vi "ScaleGenCtrl.vi"(6 "Scale Dir":T1=enum."Full scale -> Model scale", 8 "Scale factor":dbl, 11 "Gen Control (In)":T2) -> (3 "Gen Control (Out)":T2)   [LabVIEW 2018]
uses:
  Clusters/GenCtrl.ctl
  Clusters/GenMode.ctl
  Clusters/ScalingEnum.ctl
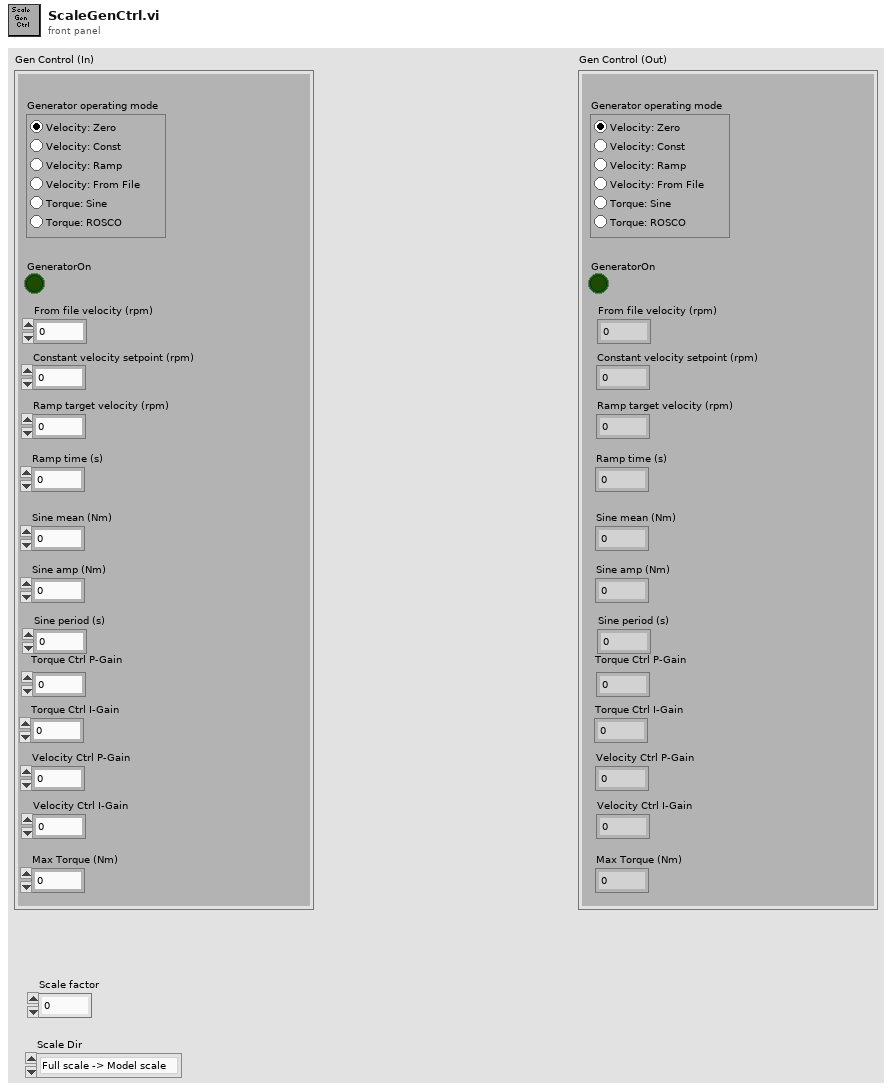
[diagram p1: front panel]
types:
  T1 = typedef "ScalingEnum.ctl" = enum16{"Model scale -> Full scale", "Full scale -> Model scale"}
  T2 = typedef "GenCtrl.ctl" = cluster{"Constant velocity setpoint (rpm)":dbl, "Ramp target velocity (rpm)":dbl, "Ramp time (s)":dbl, "Sine mean (Nm)":dbl, "Sine amp (Nm)":dbl, "Sine period (s)":dbl, "Torque Ctrl I-Gain":dbl, "Velocity Ctrl P-Gain":dbl, "Velocity Ctrl I-Gain":dbl, "Max Torque (Nm)":dbl, "GeneratorOn":bool, "Torque Ctrl P-Gain":dbl, "From file velocity (rpm)":dbl, "Generator operating mode":T3}
  T3 = typedef "GenMode.ctl" = enum32{"Velocity: Zero", "Velocity: Const.", "Velocity: Ramp", "Velocity: From File", "Torque: Sine", "Torque: ROSCO"}
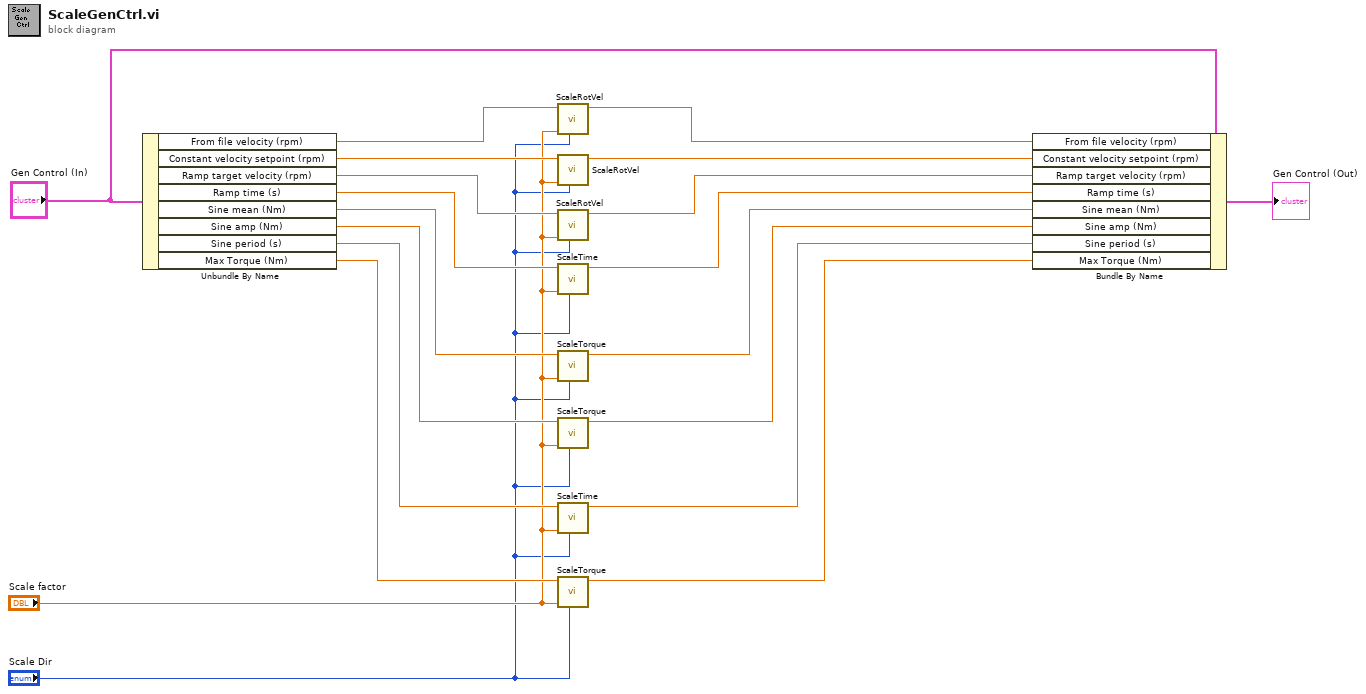
[diagram p0: block diagram]
diagram:
  n1 = Unbundle By Name("Gen Control (In)") -> ("From file velocity (rpm)"=w4:dbl, "Constant velocity setpoint (rpm)"=w18:dbl, "Ramp target velocity (rpm)"=w17:dbl, "Ramp time (s)"=w16:dbl, "Sine mean (Nm)"=w12:dbl, "Sine amp (Nm)"=w10:dbl, "Sine period (s)"=w8:dbl, "Max Torque (Nm)"=w6:dbl)
  n2 = call "ScaleRotVel.vi"("Scale Dir"="Scale Dir", "Scale factor"="Scale factor", "Rotational Velocity (In)"=w4) -> ("Rotational Velocity (Out)"=w3:dbl)  [unwired: 8 in]
  n3 = call "ScaleRotVel.vi"("Scale Dir"="Scale Dir", "Scale factor"="Scale factor", "Rotational Velocity (In)"=w18) -> ("Rotational Velocity (Out)"=w15:dbl)  [unwired: 8 in]
  n4 = call "ScaleRotVel.vi"("Scale Dir"="Scale Dir", "Scale factor"="Scale factor", "Rotational Velocity (In)"=w17) -> ("Rotational Velocity (Out)"=w14:dbl)  [unwired: 8 in]
  n5 = call "ScaleTime.vi"("Scale Dir"="Scale Dir", "Scale factor"="Scale factor", "Time (In)"=w16) -> ("Time OUT (Out)"=w13:dbl)  [unwired: 8 in]
  n6 = call "ScaleTorque.vi"("Scale Dir"="Scale Dir", "Scale factor"="Scale factor", "Torque (In)"=w12) -> ("Torque (Out)"=w11:dbl)  [unwired: 8 in]
  n7 = call "ScaleTorque.vi"("Scale Dir"="Scale Dir", "Scale factor"="Scale factor", "Torque (In)"=w10) -> ("Torque (Out)"=w9:dbl)  [unwired: 8 in]
  n8 = call "ScaleTime.vi"("Scale Dir"="Scale Dir", "Scale factor"="Scale factor", "Time (In)"=w8) -> ("Time OUT (Out)"=w7:dbl)  [unwired: 8 in]
  n9 = call "ScaleTorque.vi"("Scale Dir"="Scale Dir", "Scale factor"="Scale factor", "Torque (In)"=w6) -> ("Torque (Out)"=w5:dbl)  [unwired: 8 in]
  n10 = Bundle By Name(cluster="Gen Control (In)", "From file velocity (rpm)"=w3, "Constant velocity setpoint (rpm)"=w15, "Ramp target velocity (rpm)"=w14, "Ramp time (s)"=w13, "Sine mean (Nm)"=w11, "Sine amp (Nm)"=w9, "Sine period (s)"=w7, "Max Torque (Nm)"=w5) -> (→"Gen Control (Out)":T2)
